vi "Filter.vi"(8 "error in (no error)":errorcluster, 10 "Input":sgl[][](array[numeric]), 11 "Filter in":refnum<class "Filter.lvclass">) -> (0 "error out":errorcluster, 2 "Output":sgl[][](array[numeric]), 3 "Filter out":refnum<class "Filter.lvclass">)   [LabVIEW 2015, in "Filter.lvclass"]
uses:
  Filter.lvclass
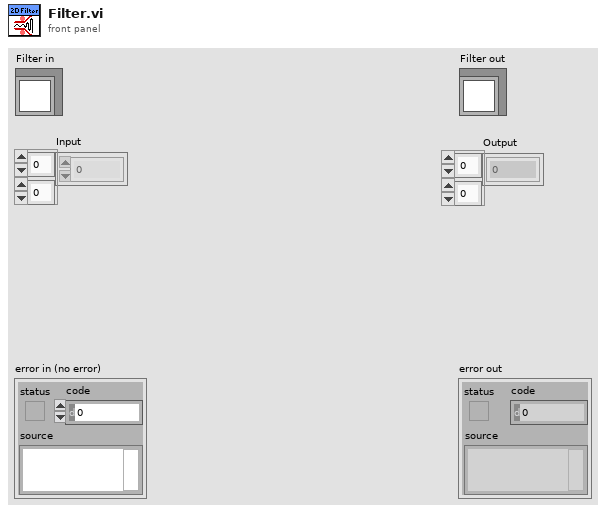
[diagram p1: front panel]
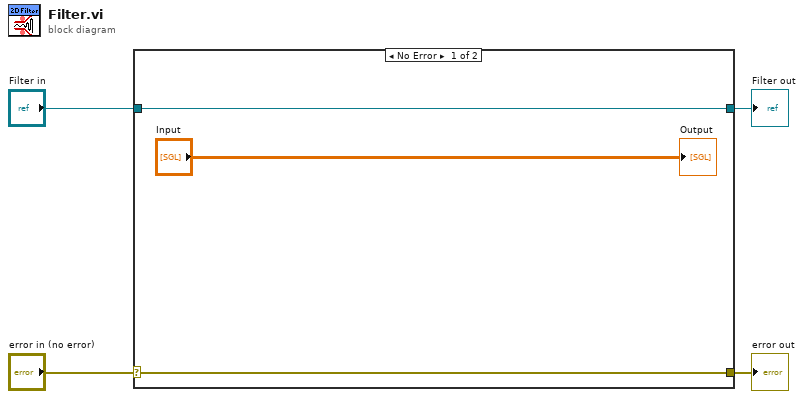
[diagram p0: block diagram]
diagram:
  n1 = case shown="No Error" "error in (no error)" {
    selector: "error in (no error)" -> [w6 w9]
    tunnel: [w6 w9] -> w3
    tunnel: [w7 w8] -> w1
    tunnel: "Filter in" -> [w7 w8]
    frame No Error {
      "Output" <- "Input"
    }
    frame Error {
    }
  }
  "error out" <- w3
  "Filter out" <- w1
